vi "SetDefaults.vi"(8 "error in (no error)":errorcluster, 11 "Logger in":refnum<class "Logger.lvclass">) -> (0 "error out":errorcluster, 3 "Logger out":refnum<class "Logger.lvclass">)   [LabVIEW 2022 SP3, in "Logger.lvlib" / "Logger.lvclass"]
uses:
  Logger.lvclass
  Logger.lvclass/Logger.ctl
  LoggingWrapper/LoggingWrapper.lvclass
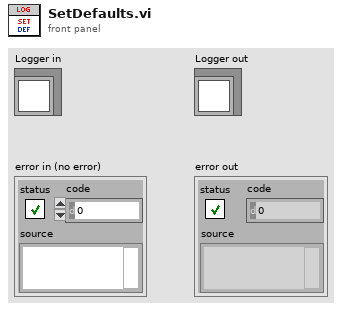
[diagram p1: front panel]
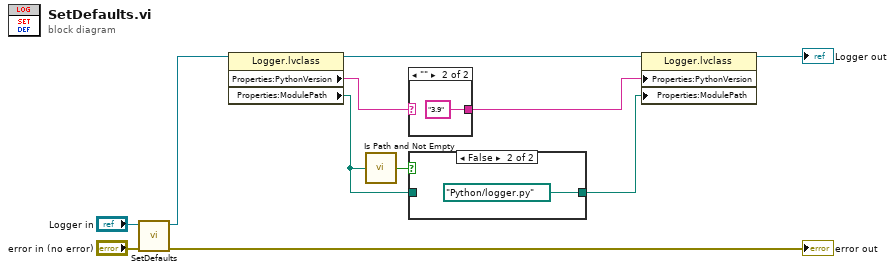
[diagram p0: block diagram]
diagram:
  n1 = call-parent "SetDefaults.vi"("error in (no error)"="error in (no error)", "PythonWrapper in"="Logger in") -> ("error out"=→"error out":errorcluster, "PythonWrapper out"=w10:refnum<class "Logger.lvclass">)  [unwired: 8 in]
  n2 = property class="Logger.lvclass"(reference=w10) -> (reference out=w7:refnum<class "Logger.lvclass">, "Properties:PythonVersion"=w5:string, "Properties:ModulePath"=w2:path)  [unwired: 1 in, 1 out]
  n3 = call <vilib>:"Is Path and Not Empty.vi"("path"=w2) -> ("Is Path and Not Empty?"=w3:bool)  [unwired: 4 in]
  n4 = case shown="\"\"" w5 {
    selector: w5 -> [w12 _]
    tunnel: [w12 "3.9"] -> w4
    frame Default {
    }
    frame "" {
    }
  }
  n5 = case shown="False" w3 {
    tunnel: [w14 path "Python/logger.py" ("Properties:ModulePath")] -> w1
    tunnel: w2 -> [w14 _]
    frame True {
    }
    frame False {
    }
  }
  n6 = property class="Logger.lvclass"(reference=w7, "Properties:PythonVersion"=w4, "Properties:ModulePath"=w1) -> (reference out=→"Logger out":refnum<class "Logger.lvclass">)  [unwired: 1 in, 1 out]
